vi "PicoScope4000aSetRapidSegments.vi"(5 "RapidBlock":bool=TRUE, 7 "nSegments":T1 format="%.4p", 8 "error in (no error)":errorcluster, 11 "handle in":i16) -> (0 "error out":errorcluster, 3 "handle out":i16, 6 "nCaptures":u64)   [LabVIEW 2010]
doc: "Calls ps5000aMemorySegments, and ps5000aSetNoOfCaptures"
uses:
  ps4000a.dll
  shared/nSegments.ctl
panel:
  out "nMaxSamples":u64
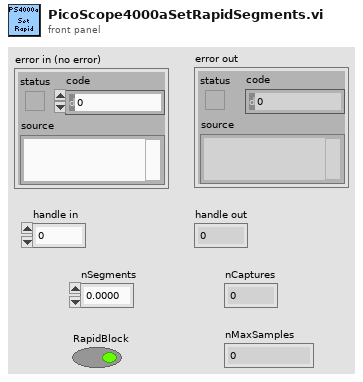
[diagram p1: front panel]
types:
  T1 = typedef "nSegments.ctl" = u64
  T2 = cluster{"status":bool, "code":u32, "source":string}
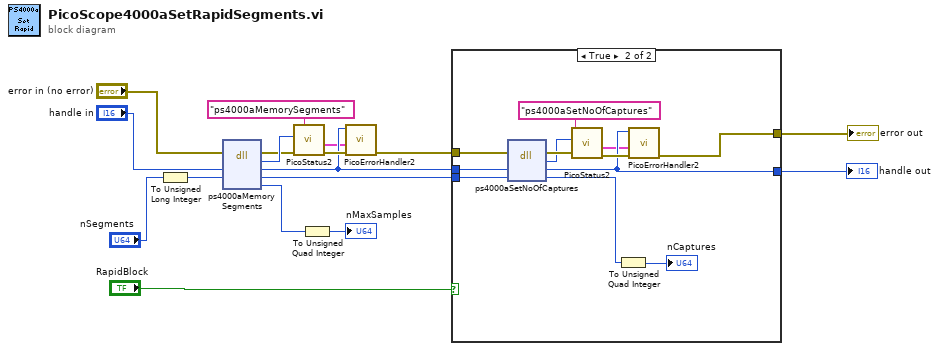
[diagram p0: block diagram]
diagram:
  n1 = To Unsigned Long Integer(number="nSegments") -> (unsigned 32bit integer=w2:u32)
  n2 = dll-call lib="ps4000a.dll" fn="ps4000aMemorySegments" ("ps3000.dll:_ps3000_open_unit@0")(error in="error in (no error)", "handle"="handle in", "nSegments"=w2) -> (error out=w16:errorcluster, "PICO_STATUS"=w17:u32, "handle"=w12:i16, "nSegments"=w14:u32, "nMaxSamples"=w4:i32)  [unwired: 3 in, 1 out]
  n3 = call "PicoStatus2.vi"("PICO source"="ps4000aMemorySegments" ("source"), "Error in"=w16, "PICO STATUS"=w17) -> ("error out"=w13:errorcluster, "PICO_STATUS out"=w1:T2)  [unwired: 5 in]
  n4 = To Unsigned Quad Integer(1:w4) -> (0:→"nMaxSamples":u64)
  n5 = call "PicoErrorHandler2.vi"("error in (no error)"=w13, "PICO_STATUS in"=w1, "handle In"=w12) -> ("error out"=w11:errorcluster)  [unwired: 8 in]
  n6 = case shown="True" "RapidBlock" {
    tunnel: w14 -> [_ w31]
    tunnel: w12 -> [w18 w28]
    tunnel: w11 -> [w19 w25]
    tunnel: [w19 w24] -> w8
    tunnel: [w18 w23] -> w7
    frame False {
    }
    frame True {
      n7 = dll-call lib="ps4000a.dll" fn="ps4000aSetNoOfCaptures" ("ps3000.dll:_ps3000_open_unit@0")(error in=w25, "handle"=w28, "nCaptures"=w31) -> (error out=w30:errorcluster, "PICO_STATUS"=w26:u32, "handle"=w23:i16, "nCaptures"=w21:u32)  [unwired: 2 in, 1 out]
      n8 = call "PicoStatus2.vi"("PICO source"="ps4000aSetNoOfCaptures" ("source"), "Error in"=w30, "PICO STATUS"=w26) -> ("error out"=w27:errorcluster, "PICO_STATUS out"=w20:T2)  [unwired: 5 in]
      n9 = To Unsigned Quad Integer(1:w21) -> (0:→"nCaptures":u64)
      n10 = call "PicoErrorHandler2.vi"("error in (no error)"=w27, "PICO_STATUS in"=w20, "handle In"=w23) -> ("error out"=w24:errorcluster)  [unwired: 8 in]
    }
  }
  "error out" <- w8
  "handle out" <- w7
